vi "Launch AC Actor.vi"(8 "error in":errorcluster, 11 "Controller in":refnum<class "Controller.lvclass">) -> (0 "error out":errorcluster, 3 "Controller out":refnum<class "Controller.lvclass">)   [LabVIEW 2014, in "Controller.lvlib" / "Controller.lvclass"]
doc: "If the <b>active?</b> flag in the configuration file associated with the aircraft network (<b>AC Network</b>) is TRUE, then this will obtain references to the configuration session and the log session and launch the <b>Network Active</b>. If the launch is successful, then this VI will return a flag stating that the launch was successful. If the launch is unsuccessful, the flag will be false and any sessions opened will be closed."
uses:
  Controller.lvclass
  Network Actor/Network Actor.lvclass
  SuperActor/SuperActor.lvclass/SuperActor.ctl
  SuperActor/Write ID.vi
  <vilib>/Utility/config.llb/Read Key (Boolean).vi
  <vilib>/Utility/config.llb/NI_LVConfig.lvlib
  SuperActor/SuperActor.lvclass
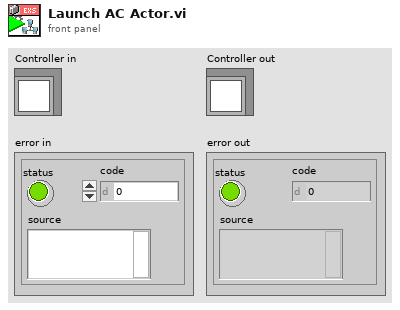
[diagram p1: front panel]
types:
  T1 = typedef "NI_LVConfig.lvlib/Config Data RefNum.ctl" = refnum<k1>
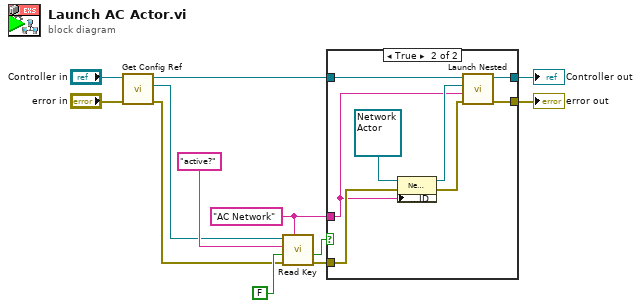
[diagram p0: block diagram]
diagram:
  w7 = "AC Network" ("section")
  n1 = call "Get Config Ref.vi"("error in"="error in", "Ex Nested in"="Controller in") -> ("error out"=w1:errorcluster, "config ref"=w5:T1, "Ex Nested out"=w3:refnum<class "Controller.lvclass">)  [unwired: 7 in]
  n2 = call-poly <vilib>:"Read Key.vi"("section"=w7, "error in (no error)"=w1, "default value"=FALSE, "key"="active?", "refnum"=w5) -> ("error out"=w6:errorcluster, "value"=w10:bool)  [unwired: 3 in, 2 out]
  n3 = case shown="True" w10 {
    tunnel: w3 -> [w13 w18]
    tunnel: [w13 w20] -> w8
    tunnel: w6 -> [w14 w21]
    tunnel: [w14 w19] -> w9
    tunnel: w7 -> [_ w16]
    frame False {
    }
    frame True {
      n4 = property class="Network Actor"(reference=refnum<class "Network Actor.lvclass"> refnum ("Network Actor Library.lvlib:Network Actor"), error in=w21, "Accessors:ID"=w16) -> (reference out=w17:refnum<class "Network Actor.lvclass">, error out=w15:errorcluster)
      n5 = call "Launch Nested.vi"("Error In"=w15, "ID"=w16, "Nested Actor"=w17, "Controller in"=w18) -> ("Error Out"=w19:errorcluster, "Controller out"=w20:refnum<class "Controller.lvclass">)  [unwired: 4 in, 2 out]
    }
  }
  "error out" <- w9
  "Controller out" <- w8
